vi "Get Uim Dev Id List wrapper.vi"(8 "error in (no error)":errorcluster caption="错误输入（无错误）", 11 "dwDevType":u32) -> (0 "error out":errorcluster caption="错误输出", 2 "devIndexList out":u32[](array[numeric]), 3 "function return":u32)   [LabVIEW 2016, in "UISimCanFunc_wrapper.lvlib"]
doc: "_declspec (dllexport) DWORD GetUimDevIdList_wrapper(DWORD dwDevType, DWORD devIndexList[]);"
uses:
  <userlib>/UISimCanFunc_wrapper/UISimCanFunc_wrapper.lvlib
  <userlib>/UISimCanFunc_wrapper/UISimCanFunc_wrapper.dll
panel:
  in  "devIndexList":u32[](array[numeric])=array[4097 elements]
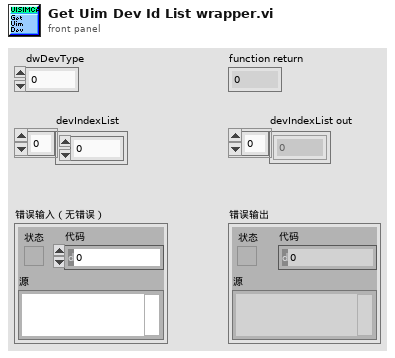
[diagram p1: front panel]
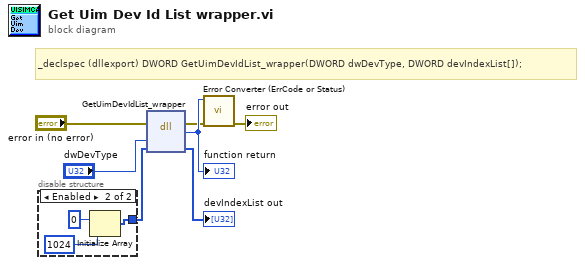
[diagram p0: block diagram]
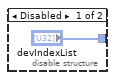
[diagram p2: hidden frame]
diagram:
  # "_declspec (dllexport) DWORD GetUimDevIdList_wrapper(DWORD dwDevType, DWORD devIndexList[]);"
  n1 = disable-structure shown="Enabled" {
    disable-tunnel: ["devIndexList" w9] -> w5
    frame Disabled {
    }
    frame Enabled {
      n2 = Initialize Array(0 ("element"), 1024 ("dimension size")) -> (w9:i32[])
    }
  }
  n3 = dll-call lib="C:/Program Files (x86)/National Instruments/LabVIEW 2016/user.lib/UISimCanFunc_wrapper/UISimCanFunc_wrapper.*" fn="GetUimDevIdList_wrapper"(error in="error in (no error)", "dwDevType"="dwDevType", "devIndexList"=w5) -> (error out=w2:errorcluster, "return type"=w7:u32, "devIndexList"=→"devIndexList out":u32[])  [unwired: 3 in, 1 out]
  "function return" <- w7
  n4 = call <userlib>:"Error Converter (ErrCode or Status).vi"("error in (no error)"=w2, "error code"=w7) -> ("error out"=→"error out":errorcluster)  [unwired: 9 in]
